vi "AddToIntegrator.vi"(10 "New samples in":u64, 11 "Integrator in":u32) -> (3 "Integrator out":u32)   [LabVIEW 2012]
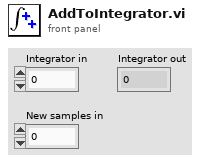
[diagram p1: front panel]
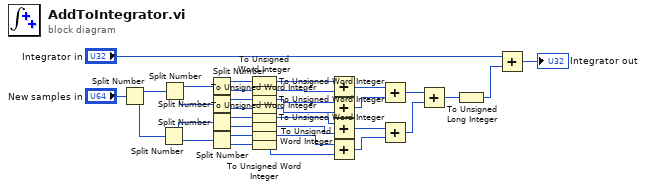
[diagram p0: block diagram]
diagram:
  n1 = Split Number(x="New samples in") -> (hi(x)=w32:u32, lo(x)=w31:u32)
  n2 = Split Number(x=w31) -> (hi(x)=w28:u16, lo(x)=w27:u16)
  n3 = Split Number(x=w32) -> (hi(x)=w30:u16, lo(x)=w29:u16)
  n4 = Split Number(x=w30) -> (hi(x)=w26:u8, lo(x)=w25:u8)
  n5 = Split Number(x=w29) -> (hi(x)=w24:u8, lo(x)=w23:u8)
  n6 = Split Number(x=w28) -> (hi(x)=w22:u8, lo(x)=w21:u8)
  n7 = Split Number(x=w27) -> (hi(x)=w20:u8, lo(x)=w19:u8)
  n8 = To Unsigned Word Integer(number=w26) -> (unsigned 16bit integer=w18:u16)
  n9 = To Unsigned Word Integer(number=w25) -> (unsigned 16bit integer=w17:u16)
  n10 = To Unsigned Word Integer(number=w24) -> (unsigned 16bit integer=w16:u16)
  n11 = To Unsigned Word Integer(number=w23) -> (unsigned 16bit integer=w15:u16)
  n12 = To Unsigned Word Integer(number=w22) -> (unsigned 16bit integer=w14:u16)
  n13 = To Unsigned Word Integer(number=w21) -> (unsigned 16bit integer=w13:u16)
  n14 = To Unsigned Word Integer(number=w20) -> (unsigned 16bit integer=w12:u16)
  n15 = To Unsigned Word Integer(number=w19) -> (unsigned 16bit integer=w11:u16)
  n16 = Add(x=w18, y=w17) -> (x+y=w10:u16)
  n17 = Add(x=w16, y=w15) -> (x+y=w9:u16)
  n18 = Add(x=w14, y=w13) -> (x+y=w8:u16)
  n19 = Add(x=w12, y=w11) -> (x+y=w7:u16)
  n20 = Add(x=w10, y=w9) -> (x+y=w5:u16)
  n21 = Add(x=w8, y=w7) -> (x+y=w6:u16)
  n22 = Add(x=w5, y=w6) -> (x+y=w4:u16)
  n23 = To Unsigned Long Integer(number=w4) -> (unsigned 32bit integer=w2:u32)
  n24 = Add(x="Integrator in", y=w2) -> (x+y=→"Integrator out":u32)
